vi "Solve General Linear Equations.vi"(2 "relative tolerance":dbl, 3 "Known Vector":dbl[](array[numeric]) format="%.2f", 4 "Input Matrix":T1) -> (0 "error":i32, 1 "Solution Vector":dbl[](array[numeric]) format="%.2f")   [LabVIEW 2017, in "NI_AALBase.lvlib"]
doc: "Solves a real linear system AX=Y using svd algorithm.\n If A is full rank, the vi finds the solution. In the case of multiple solutions, it finds the minimum 2-norm solution.\n If A is rank deficit, the vi finds the least square solution.\n\nInput Matrix is a square or rectangular, real matrix.\nKnown Vector. The number of elements in the Known Vector must be equal to the rows of the Input Matrix. If the number of elements in the Known Vector does not match the rows of the Input Matrix, the VI sets the Solution Vector to an empty array and returns an error.\n\nSolution Vector is the solution X to AX = Y.\n\nLet A be an m-by-n matrix that represents the Input Matrix, Y be the set of m coefficients in Known Vector, and X be the set of n elements in Solution Vector that solves the system AX = Y."
uses:
  NI_AALBase.lvlib
  RealMatrix.ctl
  lvanlys.dll
  NI_Matrix.lvlib
panel:
  out "Workspace":dbl[](array[numeric])
  # "Solve General Linear Equations"
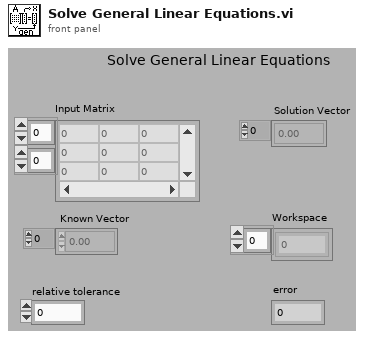
[diagram p1: front panel]
types:
  T1 = typedef "NI_Matrix.lvlib/RealMatrix.ctl" = dbl[][]
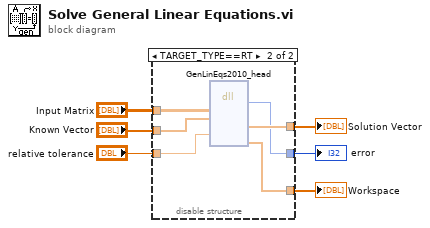
[diagram p0: block diagram]
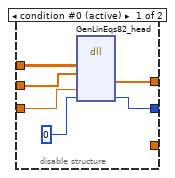
[diagram p2: hidden frame]
diagram:
  n1 = disable-structure shown="TARGET_TYPE==RT" {
    disable-tunnel: "Input Matrix" -> [w12 w18]
    disable-tunnel: "Known Vector" -> [w11 w17]
    disable-tunnel: [w10 w16] -> w4
    disable-tunnel: [w9 w14] -> w3
    disable-tunnel: "relative tolerance" -> [w7 w15]
    disable-tunnel: [_ w13] -> w1
    frame condition #0 (active) {
      n2 = dll-call lib="C:/Program Files/National Instruments/LabVIEW 2017/resource/lvanlys.*" fn="GenLinEqs82_head"("aH"=w12, "bH"=w11, "relativeTol"=w7, "dsperr"=0) -> ("xH"=w10:dbl[], "dsperr"=w9:i32)  [unwired: 8 in, 2 out]
    }
    frame condition #1 {
      n3 = dll-call lib="C:/Program Files/National Instruments/LabVIEW 2017/resource/lvanlys.*" fn="GenLinEqs2010_head" ("lvanlys.dll:GenLinEqs82_head")("aH"=w18, "bH"=w17, "relativeTol"=w15) -> ("return type"=w14:i32, "xH"=w16:dbl[], "workH"=w13:dbl[])  [unwired: 8 in, 2 out]
    }
  }
  "error" <- w3
  "Solution Vector" <- w4
  "Workspace" <- w1
